vi "resultsColumnsProfile.vi"(10 "chValuesIn":string[](array[string]), 11 "chNamesIn":string[](array[string])) -> (2 "chValuesOut":string[](array[string]), 3 "chNamesOut":string[](array[string]))   [LabVIEW 2020]
uses:
  Globals/Trav_pos_global.vi
  Globals/Meas_global.vi
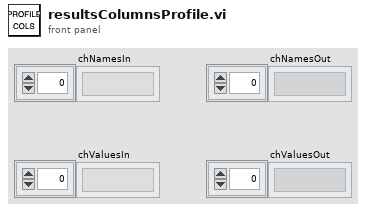
[diagram p1: front panel]
types:
  T1 = typedef "Traverse_cluster.ctl" = cluster{"Start X":sgl, "Start Y":sgl, "Start Z":sgl, "End X":sgl, "End Y":sgl, "End Z":sgl, "No. of pts.":i32, "Spacing":T2, "Filename":path, "Tunnel Speed":dbl, "Averaging time (min)":dbl, "Extra Commands":string, "Carrier_1 Q (l/min)":dbl, "Carrier_2 Q (l/min)":dbl, "Trace Gas Concentration (%)":dbl, "Specific Arguments":string, "Comments":string, "Row No":i32, "Row Type Selector":T3, "Completion time":string, "Row Duration (mins)":dbl, "No. of Valid pts.":i32, "Meas Setup File":string}
  T2 = typedef "Spacing.ctl" = enum16{"Linear", "Log", "Gauss", "Specified", "N/A"}
  T3 = typedef "Multi_run_mode.ctl" = enum16{"Move Traverse Only", "Set Tunnel Speed Only", "Set Source Only", "Set Measurement Conditions", "Single Measurement", "Vertical Profile", "Lateral Profile", "Longitudinal Profile", "Multi-Axis Profile", "Explore Volume", "Auto Calibrate", "Meas Fast FID Bkgnd", "Check Beam Power", "Scanning Valve Measurement", "Run VI Named:", "Set ADAM Ch", "Wait (minutes)", "Send Message", "Synchronize With:", "Fall Back to this Row", "Turn Off Row Repeating", "Traverse 3D Volume", "Blank Row", "Jump to Fall Back Row"}
  T4 = typedef "Post_Process.ctl" = enum16{"Take New Data", "Post Process Raw Data File"}
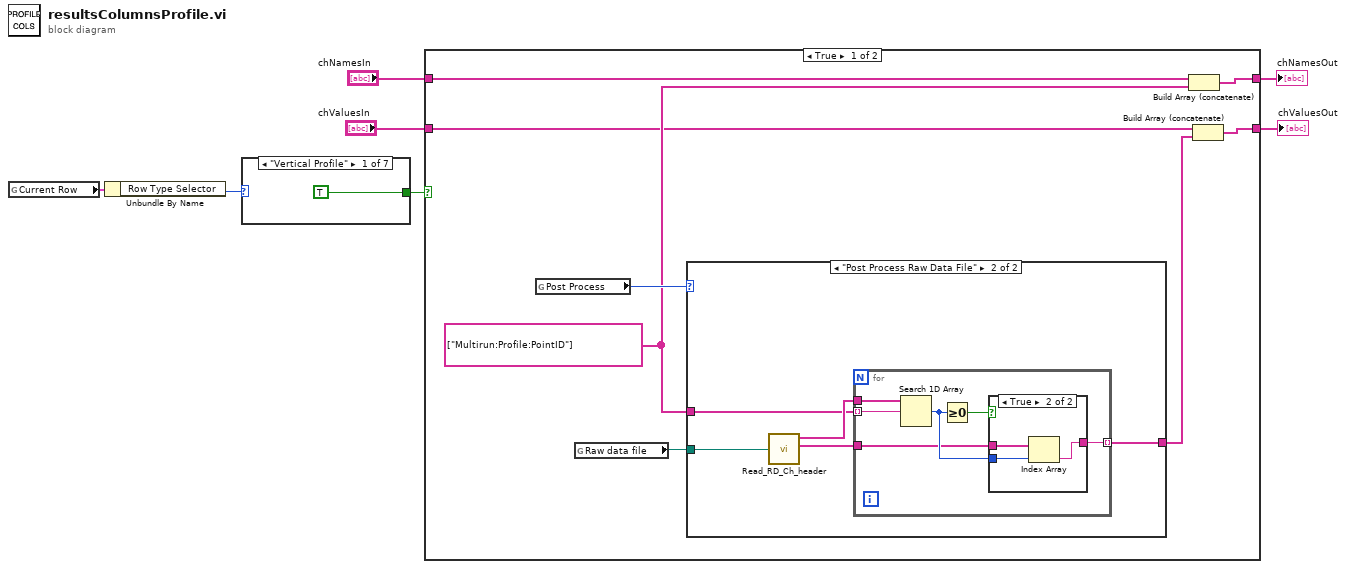
[diagram p0: block diagram]
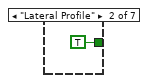
[diagram p2: hidden frame]
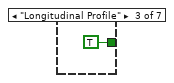
[diagram p3: hidden frame]
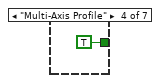
[diagram p4: hidden frame]
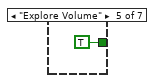
[diagram p5: hidden frame]
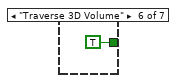
[diagram p6: hidden frame]
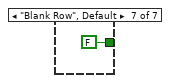
[diagram p7: hidden frame]
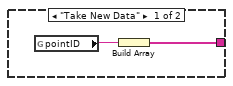
[diagram p8: hidden frame]
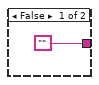
[diagram p9: hidden frame]
diagram:
  n1 = global read "Trav_pos_global.vi" "Current Row"() -> (w3:T1)
  n2 = Unbundle By Name(w3) -> ("Row Type Selector"=w2:T3)
  n3 = case shown="\"Vertical Profile\"" w2 {
    tunnel: [TRUE TRUE TRUE TRUE TRUE TRUE FALSE] -> w1
    frame "Vertical Profile" {
    }
    frame "Lateral Profile" {
    }
    frame "Longitudinal Profile" {
    }
    frame "Multi-Axis Profile" {
    }
    frame "Explore Volume" {
    }
    frame "Traverse 3D Volume" {
    }
    frame "Blank Row", Default {
    }
  }
  n4 = case shown="True" w1 {
    tunnel: [w20 w40] -> w7
    tunnel: [w19 w41] -> w6
    tunnel: "chNamesIn" -> [w16 w41]
    tunnel: "chValuesIn" -> [w15 w40]
    frame True {
      w18 = string[] ["Multirun:Profile:PointID"] ("appended array")
      n5 = global read "Meas_global.vi" "Post Process"() -> (w22:T4)
      n6 = global read "Meas_global.vi" "Raw data file"() -> (w21:path)
      n7 = case shown="\"Post Process Raw Data File\"" w22 {
        tunnel: [w23 w25] -> w17
        tunnel: w21 -> [_ w29]
        tunnel: w18 -> [_ w26]
        frame "Take New Data" {
          n8 = global read "Trav_pos_global.vi" "pointID"() -> (w24:string)
          n9 = Build Array(w24) -> (w23:string[])
        }
        frame "Post Process Raw Data File" {
          n10 = call "Read_RD_Ch_header.vi"("Raw data file"=w29) -> ("Ch Name Out"=w28:string[], "Ch Values"=w27:string[])  [unwired: 2 out]
          n11 = for {
            tunnel: w28 -> [w35]
            tunnel: w27 -> [w32]
            tunnel: [w31] -> w25 mode=indexing
            tunnel: w26 -> [w30] mode=indexing
            n12 = Search 1D Array(1D array=w35, element=w30) -> (index of element=w33:i32)  [unwired: 1 out]
            n13 = Greater Or Equal To 0?(x=w33) -> (x >= 0?=w34:bool)
            n14 = case shown="True" w34 {
              tunnel: w33 -> [_ w39]
              tunnel: w32 -> [_ w38]
              tunnel: ["" w37] -> w31
              frame False {
              }
              frame True {
                n15 = Index Array(array=w38, index=w39) -> (element=w37:string)
              }
            }
          }
        }
      }
      n16 = Build Array (concatenate)(w16, w18) -> (w19:string[])
      n17 = Build Array (concatenate)(w15, w17) -> (w20:string[])
    }
    frame False {
    }
  }
  "chValuesOut" <- w7
  "chNamesOut" <- w6
